vi "4431 Create IO Channels Simply.vi"(0 "sample mode":i32(ring)=10123 items=["Finite Samples"=10178, "Continuous Samples"=10123, "Hardware Timed Single Point"=12522], 1 "Channels: Lockin":T1={"REF f (Hz)"=[13.456], "REF phi (deg)"=[0.0]} {"REF phi (deg)" format="%#_3g"}, 6 "error in (no error)":errorcluster, 7 "AI Buffer Size (S)":i32=100, 8 "sampling info":cluster{"Fs":dbl, "#s":dbl}={"Fs"=100920.0, "#s"=7500.0}, 9 "AO":T2={"AO amp (V)"=[0.5, 0.0, 0.0, 0.0, 0.0, 0.0, 0.0, 0.0], "AO DC (V)"=[0.0, 0.0, 0.0, 0.0, 0.0, 0.0, 0.0, 0.0], "AO f (Hz)"=[13.456, 13.0, 13.0, 13.0, 13.0, 13.0, 13.0, 13.0], "AO phi (deg)"=[189.0, 0.0, 0.0, 0.0, 0.0, 0.0, 0.0, 0.0], "function"=[enum."Triangle Wave", enum."Sine Wave", enum."Sine Wave", enum."Sine Wave", enum."Sine Wave", enum."Sine Wave", enum."Sine Wave", enum."Sine Wave"]} {"AO DC (V)" format="%#_6p"; "AO amp (V)" format="%#_6p"}, 10 "AO Configuration":T3(array[cluster])=[{"Output physical channels"="Dev1/ao0", "AO. Max"=3.5, "AO.Min"=-3.5}], 11 "AI Configuration":T4(array[cluster])=[{"AI.Coupling"=enum."DC", "AI.Max"=10.0, "AI.Min"=-10.0, "Input physical channels"="Dev1/ai0:3"}]) -> (2 "AO Task":refnum<k21>[](array[refnum]), 3 "AI task":refnum<k21>[](array[refnum]), 4 "error out":errorcluster, 5 "phase log":dbl[](array[numeric])=[0.99999999999938])   [LabVIEW 2016]
uses:
  <vilib>/DAQmx/write.llb/DAQmx Write (Analog 1D Wfm NChan NSamp).vi
  <vilib>/DAQmx/read.llb/DAQmx Read (Analog 1D Wfm NChan NSamp).vi
  <vilib>/DAQmx/create/channels.llb/DAQmx Create Channel (AI-Voltage-Basic).vi
  <vilib>/DAQmx/configure/timing.llb/DAQmx Timing (Sample Clock).vi
  <vilib>/DAQmx/create/channels.llb/DAQmx Create Channel (AO-Voltage-Basic).vi
  <vilib>/DAQmx/configure/trigger.llb/DAQmx Start Trigger (Digital Edge).vi
  <vilib>/DAQmx/miscellaneous.llb/DAQmx Fill In Error Info.vi
  <resource>/objmgr/daqmx.rc
panel:
  in  "output terminal configuration":i32(ring)=-1 items=["Default"=-1, "RSE"=10083, "Differential"=10106, "Pseudodifferential"=12529]
  out "AI.FilterDelay":dbl=0.00038085937076573376
  out "AI.Gain":dbl
  in  "AI.Coupling":i32(ring)=10050 items=["AC"=10045, "DC"=10050, "GND"=10066]
  out "#samp":dbl=111.0
  in  "input terminal configuration":i32(ring)=-1 items=["default"=-1, "RSE"=10083, "NRSE"=10078, "Differential"=10106, "Pseudodifferential"=12529]
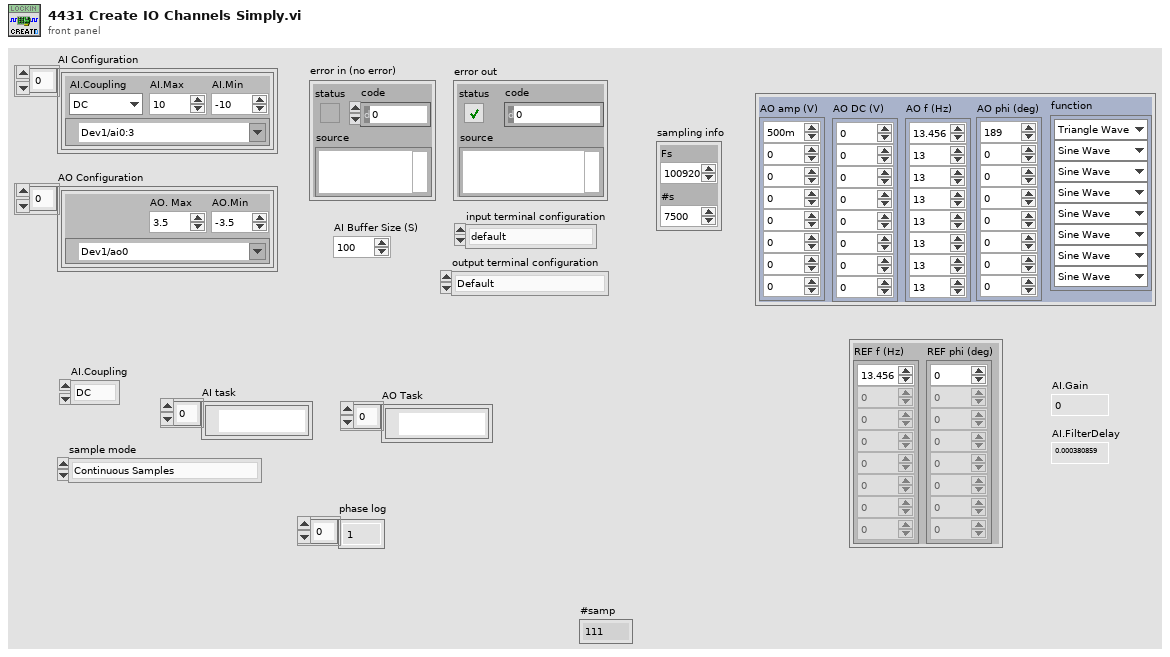
[diagram p1: front panel]
types:
  T1 = cluster{"REF f (Hz)":dbl[], "REF phi (deg)":dbl[]}
  T2 = cluster{"AO amp (V)":dbl[], "AO DC (V)":dbl[], "AO f (Hz)":dbl[], "AO phi (deg)":dbl[], "function":enum16{"Sine Wave", "Triangle Wave", "Square Wave", "Sawtooth Wave"}[]}
  T3 = cluster{"Output physical channels":tag, "AO. Max":dbl, "AO.Min":dbl}[]
  T4 = cluster{"AI.Coupling":enum16{"AC", "DC", "GND"}, "AI.Max":dbl, "AI.Min":dbl, "Input physical channels":tag}[]
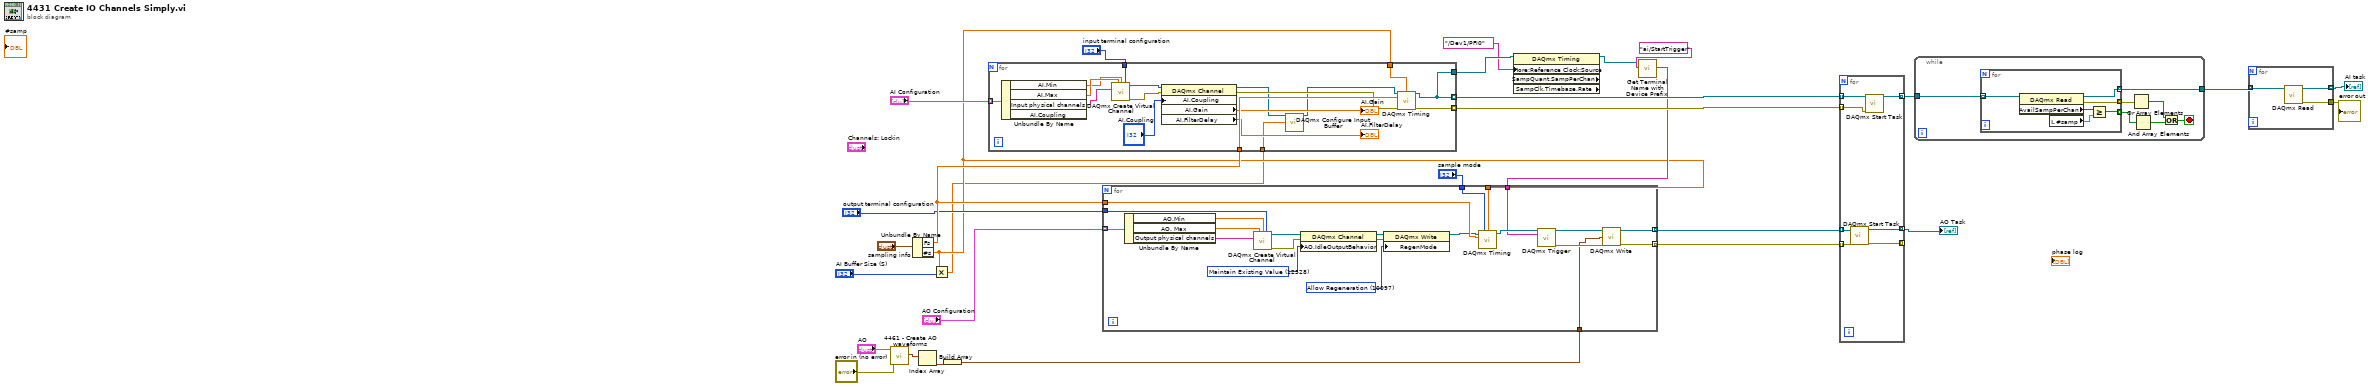
[diagram p0: block diagram]
diagram:
  n1 = call "4461 - Create AO waveforms.vi"("error in (no error)"="error in (no error)", "AO"="AO") -> ("AO Array"=w16:waveform(dbl)[])  [unwired: 6 in, 3 out]
  n2 = Unbundle By Name("sampling info") -> ("Fs"=w26:dbl, "#s"=w3:dbl)
  n3 = Index Array(array=w16) -> (element=w15:waveform(dbl))  [unwired: 1 in]
  n4 = Multiply(x=w3, y="AI Buffer Size (S)") -> (x*y=w1:dbl)
  n5 = Build Array(w15) -> (w14:waveform(dbl)[])
  n6 = for {
    tunnel: "AI Configuration" -> [w47] mode=indexing
    tunnel: w26 -> [w46]
    tunnel: "input terminal configuration" -> [w41]
    tunnel: w3 -> [w38]
    tunnel: [w36] -> w24 mode=indexing
    tunnel: [w37] -> w21 mode=indexing
    tunnel: [w36] -> w7
    tunnel: w1 -> [w32]
    n7 = Unbundle By Name(w47) -> ("AI.Min"=w42:dbl, "AI.Max"=w43:dbl, "Input physical channels"=w44:tag)  [unwired: 1 out]
    n8 = call-poly <vilib>:"DAQmx Create Virtual Channel.vi"("maximum value"=w43, "minimum value"=w42, "input terminal configuration"=w41, "physical channels"=w44) -> ("task out"=w45:refnum<k21>, "error out"=w40:errorcluster)  [unwired: 10 in]
    n9 = property class="DAQmx Channel"(reference=w45, error in=w40, "AI.Coupling"="AI.Coupling") -> (reference out=w31:refnum<k21>, error out=w39:errorcluster, "AI.Gain"=→"AI.Gain":dbl, "AI.FilterDelay"=→"AI.FilterDelay":dbl)
    n10 = call <vilib>:"DAQmx Configure Input Buffer.vi"("task/channels in"=w31, "buffer size (in samples per channel)"=w32) -> ("task out"=w30:refnum<k21>)  [unwired: 12 in, 1 out]
    n11 = call-poly <vilib>:"DAQmx Timing.vi"("task/channels in"=w30, "samples per channel"=w38, "rate"=w46, "error in"=w39) -> ("task out"=w36:refnum<k21>, "error out"=w37:errorcluster)  [unwired: 10 in]
  }
  n12 = property class="DAQmx Timing" props=["More:Reference Clock:Source", "SampQuant.SampPerChan", "SampClk.Timebase.Rate"](reference=w7, "More:Reference Clock:Source"=tag "/Dev1/PFI0" ("RefClk.Src")) -> (reference out=w5:refnum<k21>)  [unwired: 1 in, 3 out]
  n13 = call "Get Terminal Name with Device Prefix.vi"("Local Terminal Name"="ai/StartTrigger", "task/channels in"=w5) -> ("Terminal Name with Device Prefix"=w18:tag)  [unwired: 7 in, 2 out]
  n14 = for {
    tunnel: w26 -> [w60]
    tunnel: w3 -> [w58]
    tunnel: "AO Configuration" -> [w57] mode=indexing
    tunnel: w18 -> [w55]
    tunnel: w14 -> [w52]
    tunnel: "sample mode" -> [w51]
    tunnel: [w50] -> w10 mode=indexing
    tunnel: [w49] -> w9 mode=indexing
    tunnel: "output terminal configuration" -> [w48]
    w62 = 10097 items=["Allow Regeneration"=10097, "Do Not Allow Regeneration"=10158] ("RegenMode")
    w61 = 12528 items=["Zero Volts"=12526, "High-Impedance"=12527, "Maintain Existing Value"=12528] ("AO.IdleOutputBehavior")
    n15 = Unbundle By Name(w57) -> ("AO.Min"=w67:dbl, "AO. Max"=w68:dbl, "Output physical channels"=w69:tag)
    n16 = call-poly <vilib>:"DAQmx Create Virtual Channel.vi"("maximum value"=w68, "minimum value"=w67, "output terminal configuration"=w48, "physical channels"=w69) -> ("task out"=w66:refnum<k21>, "error out"=w65:errorcluster)  [unwired: 10 in]
    n17 = property class="DAQmx Channel"(reference=w66, error in=w65, "AO.IdleOutputBehavior"=w61) -> (reference out=w64:refnum<k21>, error out=w63:errorcluster)
    n18 = property class="DAQmx Write"(reference=w64, error in=w63, "RegenMode"=w62) -> (reference out=w59:refnum<k21>)  [unwired: 1 out]
    n19 = call-poly <vilib>:"DAQmx Timing.vi"("task/channels in"=w59, "sample mode"=w51, "samples per channel"=w58, "rate"=w60) -> ("task out"=w56:refnum<k21>)  [unwired: 10 in, 1 out]
    n20 = call-poly <vilib>:"DAQmx Trigger.vi"("task/channels in"=w56, "source"=w55) -> ("task out"=w54:refnum<k21>, "error out"=w53:errorcluster)  [unwired: 12 in]
    n21 = call-poly <vilib>:"DAQmx Write.vi"("task/channels in"=w54, "data"=w52, "error in"=w53) -> ("task out"=w50:refnum<k21>, "error out"=w49:errorcluster)  [unwired: 10 in, 1 out]
  }
  n22 = for {
    tunnel: w24 -> [w76] mode=indexing
    tunnel: [w75] -> w23 mode=indexing
    tunnel: w21 -> [w74] mode=indexing
    tunnel: w10 -> [w73] mode=indexing
    tunnel: w9 -> [w72] mode=indexing
    tunnel: [w71] -> _ mode=indexing
    tunnel: [w70] -> w8 mode=indexing
    n23 = call <vilib>:"DAQmx Start Task.vi"("task/channels in"=w73, "error in"=w72) -> ("task out"=w70:refnum<k21>, "error out"=w71:errorcluster)  [unwired: 12 in]
    n24 = call <vilib>:"DAQmx Start Task.vi"("task/channels in"=w76, "error in"=w74) -> ("task out"=w75:refnum<k21>)  [unwired: 12 in, 1 out]
  }
  "AO Task" <- w8
  n25 = while {
    tunnel: w23 -> [w83]
    tunnel: [w77] -> w22
    stop <- w78 stop-if-true
    n26 = for {
      tunnel: w83 -> [w89] mode=indexing
      tunnel: [w86] -> w82 mode=indexing
      tunnel: [w85] -> w81 mode=indexing
      tunnel: [w84] -> w77 mode=indexing
      n27 = property class="DAQmx Read"(reference=w89) -> (reference out=w84:refnum<k21>, error out=w86:errorcluster, "AvailSampPerChan"=w88:u32)  [unwired: 1 in]
      n28 = local read "#samp"() -> (w87:dbl)
      n29 = Greater Or Equal?(x=w88, y=w87) -> (x >= y?=w85:bool)
    }
    n30 = Or Array Elements(Boolean array=w82) -> (logical OR=w79:bool)
    n31 = And Array Elements(Boolean array=w81) -> (logical AND=w80:bool)
    n32 = Or(x=w79, y=w80) -> (x .or. y?=w78:bool)
  }
  n33 = for {
    tunnel: w22 -> [w92] mode=indexing
    tunnel: [w91] -> w20 mode=indexing
    tunnel: [w90] -> w12
    n34 = call-poly <vilib>:"DAQmx Read.vi"("task/channels in"=w92) -> ("task out"=w91:refnum<k21>, "error out"=w90:errorcluster)  [unwired: 12 in, 1 out]
  }
  "AI task" <- w20
  "error out" <- w12
